vi "Get Transformation Cluster.vi"(7 "Actual Transform In":T1, 8 "error in (no error)":errorcluster, 10 "Multiplot Representation In":T3, 11 "3D Plot.lvclass in":refnum<class "3D Plot.lvclass">) -> (0 "error out":errorcluster, 2 "Multiplot Representation Out":T3, 3 "3D Plot.lvclass out":refnum<class "3D Plot.lvclass">, 5 "Actual Transform Out":T1)   [LabVIEW 2020, in "3D Plot.lvclass"]
uses:
  <vilib>/Math Plots/3D Math Plots/3D Plot/3D Plot/3D Plot.lvclass
  <vilib>/Math Plots/3D Math Plots/3D Plot/3D Plot/Typedef/Multiplot Representation.ctl
  <vilib>/Math Plots/3D Math Plots/3D Plot/3D Plot/Typedef/Plot Representation.ctl
  <vilib>/Math Plots/3D Math Plots/3D Plot/3D Plot/Typedef/Range Clusters.ctl
  <vilib>/Math Plots/3D Math Plots/3D Plot/3D Plot/Typedef/Mesh Data.ctl
  <vilib>/Math Plots/3D Math Plots/3D Plot/3D Plot/Typedef/Actual Transform.ctl
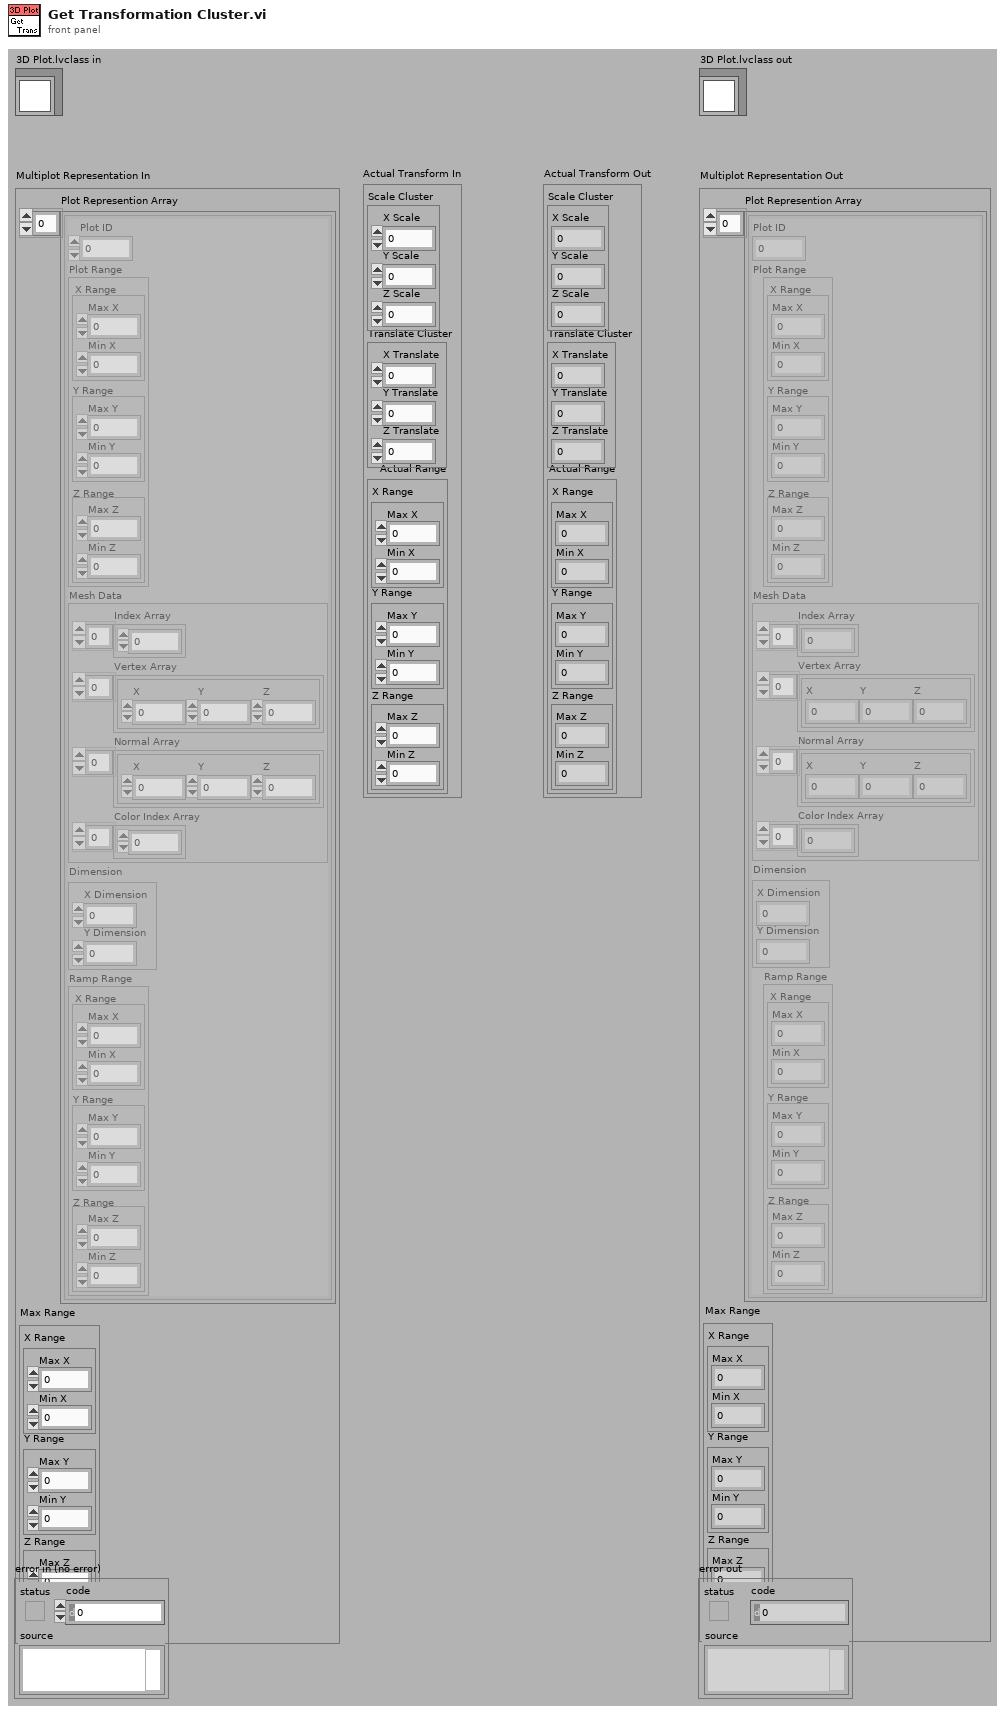
[diagram p1: front panel]
types:
  T1 = typedef "3D Plot.lvclass/Actual Transform.ctl" = cluster{"Scale Cluster":cluster{"X Scale":sgl, "Y Scale":sgl, "Z Scale":sgl}, "Translate Cluster":cluster{"X Translate":sgl, "Y Translate":sgl, "Z Translate":sgl}, "Actual Range":T2}
  T2 = typedef "3D Plot.lvclass/Range Clusters.ctl" = cluster{"X Range":cluster{"Max X":sgl, "Min X":sgl}, "Y Range":cluster{"Max Y":sgl, "Min Y":sgl}, "Z Range":cluster{"Max Z":sgl, "Min Z":sgl}}
  T3 = typedef "3D Plot.lvclass/Multiplot Representation.ctl" = cluster{"Plot Represention Array":T4[], "Max Range":T2}
  T4 = typedef "3D Plot.lvclass/Plot Representation.ctl" = cluster{"Plot ID":i32, "Plot Range":T2, "Mesh Data":T5, "Dimension":cluster{"X Dimension":i32, "Y Dimension":i32}, "Ramp Range":T2}
  T5 = typedef "3D Plot.lvclass/Mesh Data.ctl" = cluster{"Index Array":u32[], "Vertex Array":cluster{"X":sgl, "Y":sgl, "Z":sgl}[], "Normal Array":cluster{"X":sgl, "Y":sgl, "Z":sgl}[], "Color Index Array":i32[]}
  T6 = cluster{"X Range":cluster{"Max":sgl, "Min":sgl}, "Y Range":cluster{"Max":sgl, "Min":sgl}, "Z Range":cluster{"Max":sgl, "Min":sgl}}
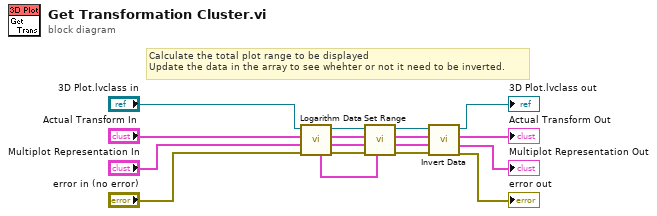
[diagram p0: block diagram]
diagram:
  # "Calculate the total plot range to be displayed\nUpdate the data in the array to see whehter or not it need to be inverted."
  n1 = call <vilib>:"Logarithm Data.vi"("error in (no error)"="error in (no error)", "Multiplot Representation In"="Multiplot Representation In", "Actual Transform In"="Actual Transform In", "3D Plot.lvclass in"="3D Plot.lvclass in") -> ("error out"=w8:errorcluster, "Multiplot Representation In"=w7:T3, "Actual Transform Out"=w6:T1, "3D Plot.lvclass out"=w4:refnum<class "3D Plot.lvclass">, "Range Cluster"=w3:T6)  [unwired: 1 in, 2 out]
  n2 = call <vilib>:"Set Range.vi"("Range Cluster"=w3, "error in (no error)"=w8, "Multiplot Representation In"=w7, "Actual Transform In"=w6, "3D Plot.lvclass in"=w4) -> ("error out"=w16:errorcluster, "Multiplot Representation In"=w15:T3, "Actual Transform Out"=w17:T1, "3D Plot.lvclass out"=w2:refnum<class "3D Plot.lvclass">)  [unwired: 3 out]
  n3 = call-dynamic "Invert Data.vi"("error in (no error)"=w16, "Multiplot Representation In"=w15, "Actual Transform In"=w17, "3D Plot.lvclass in"=w2) -> ("error out"=→"error out":errorcluster, "Multiplot Representation In"=→"Multiplot Representation Out":T3, "Actual Transform Out"=→"Actual Transform Out":T1, "3D Plot.lvclass out"=→"3D Plot.lvclass out":refnum<class "3D Plot.lvclass">)  [unwired: 4 out]
